vi "Get VI name.vi"(11 "VI in":refnum<vi>) -> (1 "Full Vi Name":string, 2 "Plain Name":string, 3 "VI out":refnum<vi>)   [LabVIEW 2019, in "Panther Dashboard.lvlib"]
uses:
  Panther Dashboard.lvlib
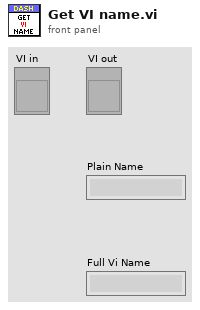
[diagram p1: front panel]
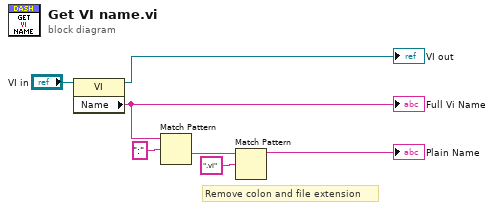
[diagram p0: block diagram]
diagram:
  # "Remove colon and file extension"
  n1 = property class="VI"(reference="VI in") -> (reference out=→"VI out":refnum<vi>, "Name"=w6:string)  [unwired: 1 in, 1 out]
  "Full Vi Name" <- w6
  n2 = Match Pattern(string=w6, regular expression=":") -> (after substring=w3:string)  [unwired: 1 in, 3 out]
  n3 = Match Pattern(string=w3, regular expression=".vi") -> (before substring=→"Plain Name":string)  [unwired: 1 in, 3 out]
